vi "ReadMultiDriveCounters.vi"(0 "Recheck if Moved?":bool, 1 "Position input XYZ":sgl[](array[numeric])=[0.0, 0.0, 0.0] format="%.2f", 2 "Channel Properties":T1[](array[typedef]) {"Current Pos" format="%.2f"; "Backlash/Eng units" format="%.2f"; "Pulses/rev" format="%.2f"; "Pos Tolerance" format="%.2f"; "Pulses/unit" format="%.2f"; "Acc. Min" format="%.2f"; "Acc. Max" format="%.2f"; "Vel. Min" format="%.2f"; "Vel. Max" format="%.2f"; "Acc. Default" format="%.2f"; "Vel. Default" format="%.2f"}) -> (3 "Pulses":sgl[](array[numeric]), 4 "Eng units":sgl[](array[numeric]) format="%.2f", 5 "Position Correct":bool, 6 "Error String":string)   [LabVIEW 2022 SP3]
uses:
  GenericDriveCommand.ctl
  Anemometry/Anemometry Sub Vis/Controls/In_Range.ctl
  Anemometry/Anemometry Sub Vis/Globals/Trav_pos_global.vi
  DriveProperties.ctl
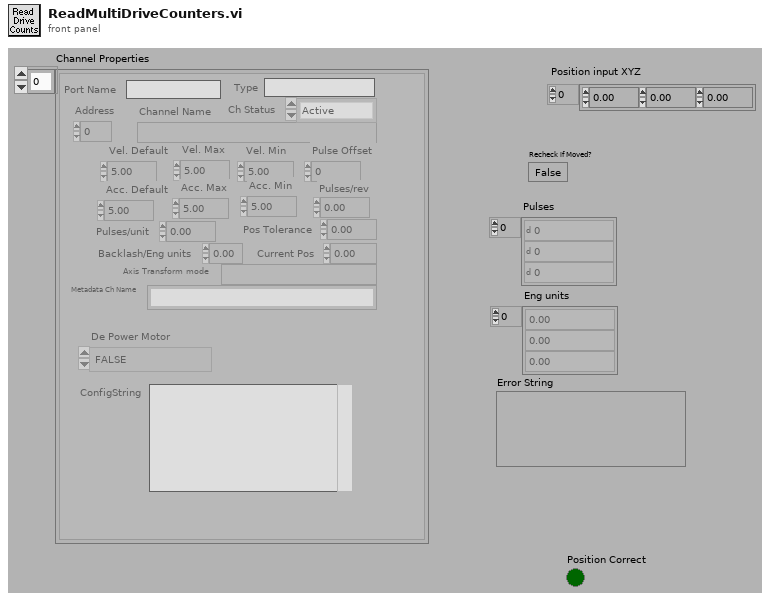
[diagram p1: front panel]
types:
  T1 = typedef "DriveProperties.ctl" = cluster{"Channel Name":string, "Vel. Default":sgl, "Acc. Default":sgl, "Vel. Max":sgl, "Vel. Min":sgl, "Acc. Max":sgl, "Acc. Min":sgl, "Pulses/unit":sgl, "Address":u8, "Pulse Offset":i32, "Pos Tolerance":sgl, "Pulses/rev":sgl, "Backlash/Eng units":sgl, "Current Pos":sgl, "Ch Status":enum16{"Active", "Offline", "Simulate"}, "Port Name":string, "Axis Transform mode":string, "Metadata Ch Name":string, "Type":string, "De Power Motor":enum16{"TRUE", "FALSE"}, "ConfigString":string}
  T2 = typedef "GenericDriveCommand.ctl" = string
  T3 = typedef "In_Range.ctl" = enum16{"%", "±", "% & ±"}
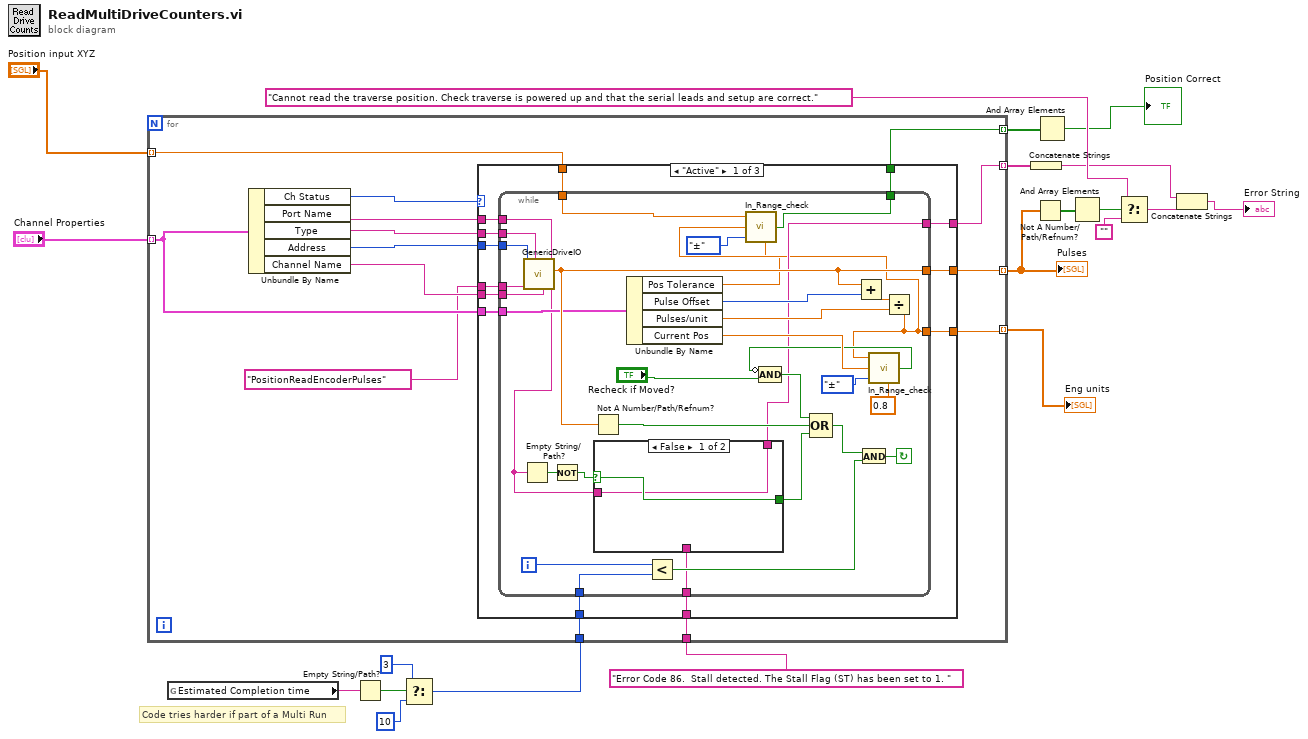
[diagram p0: block diagram]
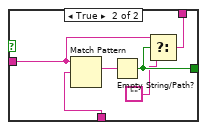
[diagram p2: hidden frame]
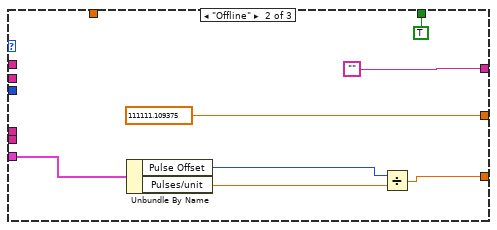
[diagram p3: hidden frame]
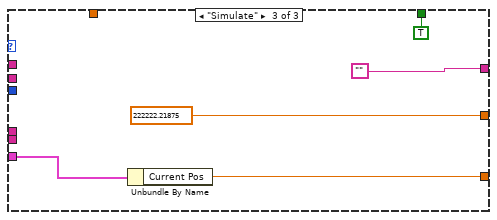
[diagram p4: hidden frame]
diagram:
  # "Code tries harder if part of a Multi Run"
  n1 = global read "Trav_pos_global.vi" "Estimated Completion time"() -> (w10:string)
  n2 = Empty String/Path?(string/path=w10) -> (empty?=w9:bool)
  n3 = Select(t=3, s=w9, f=10) -> (s? t:f=w6:i32)
  n4 = for {
    tunnel: [w34] -> w19 mode=indexing
    tunnel: "Channel Properties" -> [w31] mode=indexing
    tunnel: [w30] -> w20 mode=indexing
    tunnel: [w26] -> w14 mode=indexing
    tunnel: w6 -> [w25]
    tunnel: "Error Code 86.  Stall detected. The Stall Flag (ST) has been set to 1. " -> [w24]
    tunnel: "Position input XYZ" -> [w23] mode=indexing
    tunnel: [w22] -> w3 mode=indexing
    n5 = Unbundle By Name(w31) -> ("Ch Status"=w29:enum16{"Active", "Offline", "Simulate"}, "Port Name"=w32:string, "Type"=w28:string, "Address"=w33:u8, "Channel Name"=w27:string)
    n6 = case shown="\"Active\"" w29 {
      tunnel: T2 "PositionReadEncoderPulses" ("GenericDriveCommand") -> [w47 _ _]
      tunnel: w33 -> [w46 _ _]
      tunnel: [w45 sgl 111111.11 ("Numeric Reply") sgl 222222.22 ("Numeric Reply")] -> w34
      tunnel: w28 -> [w44 _ _]
      tunnel: w32 -> [w43 _ _]
      tunnel: w31 -> [w42 w95 w100]
      tunnel: [w41 w91 w98] -> w30
      tunnel: w27 -> [w40 _ _]
      tunnel: [w39 "" ""] -> w26
      tunnel: w25 -> [w38 _ _]
      tunnel: w24 -> [w37 _ _]
      tunnel: w23 -> [w36 _ _]
      tunnel: [w35 TRUE ("In Range") TRUE ("In Range")] -> w22
      frame "Active" {
        n7 = while {
          tunnel: [w52] -> w41
          tunnel: w42 -> [w73]
          tunnel: w43 -> [w78]
          tunnel: w44 -> [w67]
          tunnel: [w74] -> w45
          tunnel: w46 -> [w79]
          tunnel: w47 -> [w80]
          tunnel: w40 -> [w66]
          tunnel: [w53] -> w39
          tunnel: w38 -> [w60]
          tunnel: w37 -> [w54]
          tunnel: w36 -> [w51]
          tunnel: [w48] -> w35
          i -> [w61]
          stop <- w65 continue-if-true
          n8 = call "GenericDriveIO.vi"("GenericDriveCommand"=w80, "Channel Name"=w66, "Address"=w79, "Type"=w67, "Port Name"=w78) -> ("Error Description"=w57:string, "Numeric Reply"=w74:sgl)  [unwired: 1 in, 4 out]
          n9 = Empty String/Path?(string/path=w57) -> (empty?=w58:bool)
          n10 = Not(x=w58) -> (.not. x?=w56:bool)
          n11 = Not A Number/Path/Refnum?(number/path/refnum=w74) -> (NaN/Path/Refnum?=w63:bool)
          n12 = case shown="False" w56 {
            selector: w56 -> [w82 _]
            tunnel: [w82 w86] -> w55
            tunnel: w57 -> [w81 w85]
            tunnel: w54 -> [_ w87]
            tunnel: [w81 w84] -> w53
            frame False {
            }
            frame True {
              n13 = Match Pattern(string=w85, regular expression=w87) -> (match substring=w88:string)  [unwired: 1 in, 3 out]
              n14 = Empty String/Path?(string/path=w88) -> (empty?=w86:bool)
              n15 = Select(t=w85, s=w86, f="") -> (s? t:f=w84:string)
            }
          }
          n16 = Unbundle By Name(w73) -> ("Pos Tolerance"=w49:sgl, "Pulse Offset"=w76:i32, "Pulses/unit"=w77:sgl, "Current Pos"=w72:sgl)
          n17 = Less?(x=w61, y=w60) -> (x < y?=w59:bool)
          n18 = Add(x=w74, y=w76) -> (x+y=w75:sgl)
          n19 = Divide(x=w75, y=w77) -> (x/y=w52:sgl)
          n20 = call "In_Range_check.vi"("±"=w49, "Mode"=In_Range."±", "Value"=w52, "Setpoint"=w51) -> ("In Range"=w48:bool)  [unwired: 1 in, 2 out]
          n21 = call "In_Range_check.vi"("±"=0.8, "Mode"=In_Range."±", "Value"=w72, "Setpoint"=w52) -> ("In Range"=w69:bool)  [unwired: 1 in, 2 out]
          n22 = Compound Arithmetic op=AND(invert w69, "Recheck if Moved?") -> (w64:bool)
          n23 = Compound Arithmetic op=OR(w64, w63, w55) -> (w62:bool)
          n24 = And(x=w62, y=w59) -> (x .and. y?=w65:bool)
        }
      }
      frame "Offline" {
        n25 = Unbundle By Name(w95) -> ("Pulse Offset"=w93:i32, "Pulses/unit"=w92:sgl)
        n26 = Divide(x=w93, y=w92) -> (x/y=w91:sgl)
      }
      frame "Simulate" {
        n27 = Unbundle By Name(w100) -> ("Current Pos"=w98:sgl)
      }
    }
  }
  "Pulses" <- w19
  "Eng units" <- w20
  n28 = Concatenate Strings(w14) -> (w11:string)
  n29 = Not A Number/Path/Refnum?(number/path/refnum=w19) -> (NaN/Path/Refnum?=w18:bool[])
  n30 = And Array Elements(Boolean array=w3) -> (logical AND=→"Position Correct":bool)
  n31 = And Array Elements(Boolean array=w18) -> (logical AND=w17:bool)
  n32 = Select(t="Cannot read the traverse position. Check traverse is powered up and that the serial leads and setup are correct.", s=w17, f="") -> (s? t:f=w13:string)
  n33 = Concatenate Strings(w11, w13) -> (→"Error String":string)
